vi "Initialize.vi"(8 "error in":errorcluster, 11 "VISA resource name":refnum<visa-resource-name>) -> (0 "error out":errorcluster, 3 "VISA resource name out":refnum<visa-resource-name>)   [LabVIEW 2020]
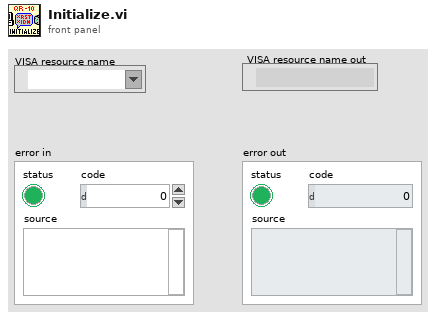
[diagram p1: front panel]
types:
  T1 = cluster{"Baud Rate":u32, "Parity":u16, "Data Bits":u16, "Stop Bits":u16, "Flow Control":u16}
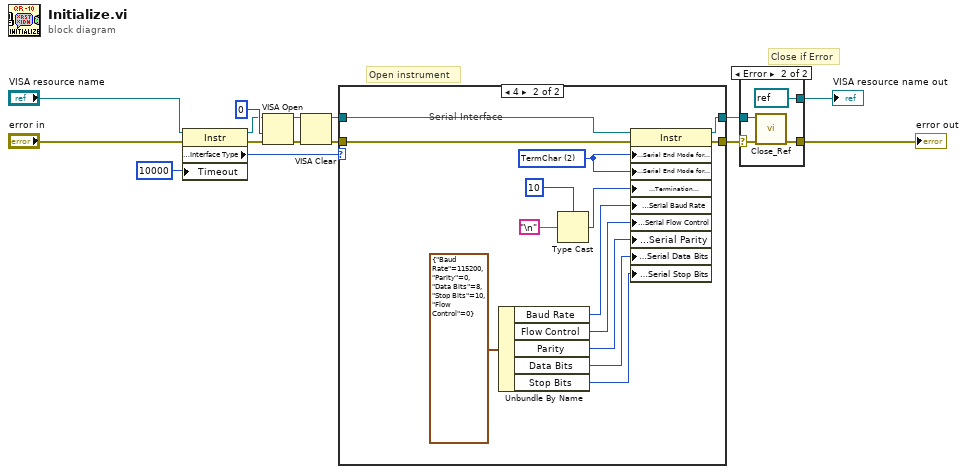
[diagram p0: block diagram]
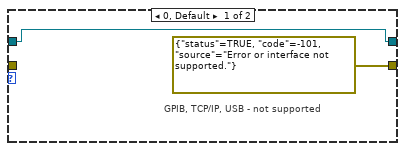
[diagram p2: hidden frame]
diagram:
  # "Close if Error"
  # "Open instrument"
  n1 = property class="Instr"(reference="VISA resource name", error in="error in", "Timeout"=u32 10000 ("General Settings:Timeout Value")) -> (reference out=w7:refnum<visa-resource-name>, error out=w5:errorcluster, "Interface Information:Interface Type"=w11:u16)
  n2 = VISA Open(access mode=u32 0, error in (no error)=w5, VISA resource name=w7) -> (VISA resource name=w8:refnum<visa-resource-name>, error out=w9:errorcluster)  [unwired: 2 in]
  n3 = VISA Clear(VISA resource name=w8, error in (no error)=w9) -> (VISA resource name out=w6:refnum<visa-resource-name>, error out=w4:errorcluster)
  n4 = case shown="4" w11 {
    tunnel: [w17 w30] -> w15
    tunnel: [errorcluster {"status"=TRUE, "code"=-101, "source"="Error or interface not supported."} ("error out") w31] -> w14
    tunnel: w4 -> [_ w18]
    tunnel: w6 -> [w17 w19]
    frame 0, Default {
      # "GPIB, TCP/IP, USB - not supported"
    }
    frame 4 {
      w27 = u16 2 items=["None", "LastBit", "TermChar"] ("Serial Settings:Serial End Mode for Reads")
      # "Serial Interface"
      n5 = Unbundle By Name(T1 {"Baud Rate"=115200, "Parity"=0, "Data Bits"=8, "Stop Bits"=10, "Flow Control"=0} ("Serial Configuration")) -> ("Baud Rate"=w25:u32, "Flow Control"=w21:u16, "Parity"=w23:u16, "Data Bits"=w24:u16, "Stop Bits"=w20:u16)
      n6 = Type Cast(type=u8 10, x="\n" ("Line Feed Constant")) -> (*(type *) &x=w26:u8)
      n7 = property class="Instr"(reference=w19, error in=w18, "Serial Settings:Serial End Mode for Reads"=w27, "Serial Settings:Serial End Mode for Writes"=w27, "Message Based Settings:Termination Character"=w26, "Serial Settings:Serial Baud Rate"=w25, "Serial Settings:Serial Flow Control"=w21, "Serial Settings:Serial Parity"=w23, "Serial Settings:Serial Data Bits"=w24, "Serial Settings:Serial Stop Bits"=w20) -> (reference out=w30:refnum<visa-resource-name>, error out=w31:errorcluster)
    }
  }
  n8 = case shown="Error" w14 {
    selector: w14 -> [w32 w35]
    tunnel: w15 -> [w33 w36]
    tunnel: [w33 refnum<visa-resource-name> refnum ("VISA resource name out")] -> w13
    tunnel: [w32 w34] -> w2
    frame No Error {
    }
    frame Error {
      n9 = call "Close_Ref.vi"("error in"=w35, "VISA resource name"=w36) -> ("error out"=w34:errorcluster)  [unwired: 9 in]
    }
  }
  "VISA resource name out" <- w13
  "error out" <- w2
